vi "Calculate Placing Accuracy.vi"() -> ()   [LabVIEW 2017]
uses:
  Shared Components/Gantry Class/Type Definitions/Virtual Modes.ctl
  Shared Components/Gantry Class/Type Definitions/Init_Modes.ctl
  Shared Components/Utils/Type Definitions/Object Types.ctl
  Shared Components/Config Manager Class/Type Definitions/Camera Enum.ctl
  Shared Components/Gantry Class/Gantry Class.lvclass
  Shared Components/Vec3d Class/Vec3d Class.lvclass
panel:
  in  "Results Folder":path=path "C:/Users/Admin/Gantry Purdue/pixel-gantry-control/Results"
  out "Point being recorded":string="\\P"
  out "Iteration Number":i32
  in  "Virtual Mode":T1=enum."Virtual"
  in  "stop":bool
  out "Image":T2(plugin-control)
  out "error out":errorcluster
  in  "Config Folder":path=path "C:/Users/Admin/Gantry Purdue/pixel-gantry-control/Config"
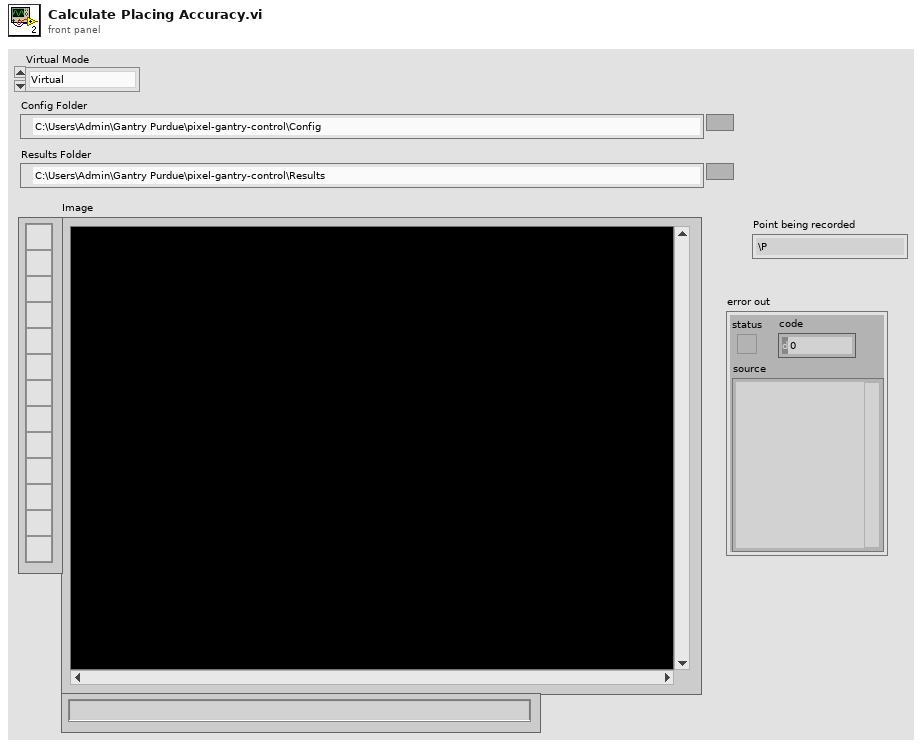
[diagram p1: front panel]
types:
  T1 = typedef "Virtual Modes.ctl" = enum16{"Nonvirtual", "Pseudovirtual", "Virtual"}
  T2 = typedef "IMAQ Image.ctl" = refnum<image>
  T3 = typedef "Init_Modes.ctl" = enum16{"Full", "Robot Only", "Dispenser Only", "Cameras Only", "Robot and Cameras", "Robot and Cameras and Dispenser", "Manifold Only"}
  T4 = typedef "Object Types.ctl" = enum16{"HDI", "Glass Piece", "Other"}
  T5 = typedef "Camera Enum.ctl" = enum16{"GANTRY HEAD", "NEEDLE CALIBRATION X", "NEEDLE CALIBRATION Y", "STAND CAMERA", "SIMRAN WEBCAM"}
  T6 = typedef "Physical Image.ctl" = cluster{"Image Position":refnum<class "Vec3d Class.lvclass">, "Image Reference":T2, "Field of View":cluster{"x(mm)":dbl, "y(mm)":dbl}}
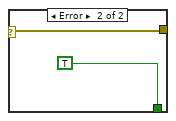
[diagram p2: hidden frame]
diagram:
  n1 = property on="stop" class="Bool (strict)"("Value"=FALSE) -> (error out=w14:errorcluster)  [unwired: 2 in, 1 out]
  n2 = call "IMAQ Create"("Image Name"="test") -> ("New Image"=w11:T2)  [unwired: 4 in, 1 out]
  n3 = property on="error out" class="Clust (strict)"(error in=w14, "Value"=errorcluster {"status"=FALSE, "code"=0, "source"=""} ("error in (no error)")) -> (error out=w9:errorcluster)  [unwired: 1 in, 1 out]
  n4 = call "Create.vi"("Virtual Mode"="Virtual Mode", "error in"=w9, "HOME?"=TRUE, "Config Folder"="Config Folder", "Init Mode"=Init_Modes."Full") -> ("error out"=w6:errorcluster, "Gantry out"=w5:refnum<class "Gantry Class.lvclass">)  [unwired: 5 in]
  n5 = while {
    shift-right: [w72] -> w3
    shift-left: w11 -> [w122]
    shift-right: [w124] -> w2
    shift-left: w5 -> [w158]
    shift-right: [w123] -> w1
    shift-left: w6 -> [w163]
    i -> [w160]
    stop <- w161 stop-if-true
    # "INSERT ROTATION OF STATION"
    # "INSERT MIDPT OF STATION"
    # "Pick up tool"
    # "Return tool"
    n6 = call "HDI fiducials"("error in (no error)"=w163) -> ("error out"=w156:errorcluster)  [unwired: 17 in, 1 out]
    n7 = call-dynamic "Set Manifold Channel.vi"("error in"=w156, "On/Off"=TRUE, "Manifold Channel"=29, "Gantry in"=w158) -> ("error out"=w155:errorcluster, "Gantry out"=w157:refnum<class "Gantry Class.lvclass">)  [unwired: 6 in]
    n8 = call "Create.vi"("error in"=w155, "Z"=30.0, "Y"=193.8, "X"=549.36) -> ("error out"=w243:errorcluster, "Vec3d Class out"=w276:refnum<class "Vec3d Class.lvclass">)  [unwired: 6 in]
    n9 = call-dynamic "Move To Raw.vi"("error in"=w243, "Speed"=80.0, "Destination"=w276, "Gantry in"=w157) -> ("error out"=w63:errorcluster, "Gantry out"=w68:refnum<class "Gantry Class.lvclass">)  [unwired: 6 in]
    n10 = call "Create.vi"("error in"=w63, "Z"=57.76) -> ("error out"=w62:errorcluster, "Vec3d Class out"=w69:refnum<class "Vec3d Class.lvclass">)  [unwired: 8 in]
    n11 = call-dynamic "Move To Raw Relative.vi"("error in"=w62, "Speed(mm/s)"=10.0, "Delta"=w69, "Gantry in"=w68) -> ("error out"=w66:errorcluster, "Gantry out"=w67:refnum<class "Gantry Class.lvclass">)  [unwired: 6 in]
    n12 = call-dynamic "Midpt&Orient.vi"("error in (no error)"=w66, "Enum"=Object_Types."Glass Piece", "Image In"=w122, "Gantry Class in"=w67) -> ("error out"=w176:errorcluster, "Midpoint"=w241:refnum<class "Vec3d Class.lvclass">, "Image Out"=w25:T2, "Gantry Class out"=w168:refnum<class "Gantry Class.lvclass">, "Orientation"=w165:dbl)  [unwired: 3 in]
    n13 = call "Create.vi"("error in"=w176, "Z"=34.374944 ("Y"), "Y"=-101.797103, "X"=-0.484739) -> ("error out"=w169:errorcluster, "Vec3d Class out"=w214:refnum<class "Vec3d Class.lvclass">)  [unwired: 6 in]
    n14 = call-dynamic "Home Single.vi"("error in"=w169, "Axis"=enum16{"X", "Y", "Z", "U"}."Z", "Gantry in"=w168) -> ("error out"=w166:errorcluster, "Gantry out"=w167:refnum<class "Gantry Class.lvclass">)  [unwired: 7 in]
    n15 = call "Create.vi"("error in"=w166, "Y"=16.37, "X"=603.594) -> ("Vec3d Class out"=w292:refnum<class "Vec3d Class.lvclass">)  [unwired: 7 in, 1 out]
    n16 = call-dynamic "Move To Raw.vi"("Speed"=50.0 ("Speed(mm/s)"), "Destination"=w292, "Gantry in"=w167) -> ("error out"=w188:errorcluster, "Gantry out"=w189:refnum<class "Gantry Class.lvclass">)  [unwired: 7 in]
    n17 = call "Create.vi"("Z"=36.7) -> ("Vec3d Class out"=w190:refnum<class "Vec3d Class.lvclass">)  [unwired: 9 in, 1 out]
    n18 = call-dynamic "Move To Raw Relative.vi"("error in"=w188, "Speed(mm/s)"=10.0, "Delta"=w190, "Gantry in"=w189) -> ("error out"=w52:errorcluster, "Gantry out"=w51:refnum<class "Gantry Class.lvclass">)  [unwired: 6 in]
    n19 = call-dynamic "Set Manifold Channel.vi"("error in"=w52, "On/Off"=TRUE, "Manifold Channel"=0, "Gantry in"=w51) -> ("error out"=w54:errorcluster, "Gantry out"=w56:refnum<class "Gantry Class.lvclass">)  [unwired: 6 in]
    n20 = call "Create.vi"("Z"=4.5) -> ("Vec3d Class out"=w57:refnum<class "Vec3d Class.lvclass">)  [unwired: 9 in, 1 out]
    n21 = call-dynamic "Move To Raw Relative.vi"("error in"=w54, "Speed(mm/s)"=1.0, "Delta"=w57, "Gantry in"=w56) -> ("error out"=w53:errorcluster, "Gantry out"=w55:refnum<class "Gantry Class.lvclass">)  [unwired: 6 in]
    n22 = flat-sequence {
      tunnel: w55 -> [w380]
      tunnel: [w380] -> w250
      tunnel: w53 -> [w378]
      tunnel: [w378] -> w249
      frame #0 {
        n23 = Wait (ms)(milliseconds to wait=u32 1000) -> ()  [unwired: 1 out]
      }
    }
    n24 = call "Create.vi"("Z"=-4.5) -> ("Vec3d Class out"=w287:refnum<class "Vec3d Class.lvclass">)  [unwired: 9 in, 1 out]
    n25 = call-dynamic "Move To Raw Relative.vi"("Wait?"=TRUE, "error in"=w249, "Speed(mm/s)"=1.0, "Delta"=w287, "Gantry in"=w250) -> ("error out"=w282:errorcluster, "Gantry out"=w283:refnum<class "Gantry Class.lvclass">)  [unwired: 5 in]
    n26 = call "Create.vi"("Y"=80.0 ("Z")) -> ("Vec3d Class out"=w281:refnum<class "Vec3d Class.lvclass">)  [unwired: 9 in, 1 out]
    n27 = call-dynamic "Move To Raw Relative.vi"("error in"=w282, "Speed(mm/s)"=10.0, "Delta"=w281, "Gantry in"=w283) -> ("error out"=w269:errorcluster, "Gantry out"=w271:refnum<class "Gantry Class.lvclass">)  [unwired: 6 in]
    n28 = call-dynamic "Get Current Position Raw.vi"("error in"=w269, "Gantry in"=w271) -> ("error out"=w268:errorcluster, "Vec3d Class out"=w205:refnum<class "Vec3d Class.lvclass">, "Gantry out"=w270:refnum<class "Gantry Class.lvclass">)  [unwired: 7 in]
    n29 = call "Create.vi"("Z"=-36.7) -> ("Vec3d Class out"=w277:refnum<class "Vec3d Class.lvclass">)  [unwired: 9 in, 1 out]
    n30 = call-dynamic "Move To Raw Relative.vi"("error in"=w268, "Speed(mm/s)"=10.0, "Delta"=w277, "Gantry in"=w270) -> ("error out"=w235:errorcluster, "Gantry out"=w233:refnum<class "Gantry Class.lvclass">)  [unwired: 6 in]
    n31 = call "Subtract Vec3d.vi"("error in (no error)"=w235, "Vec3d in 2"=w214, "Vec3d in 1"=w241) -> ("error out"=w237:errorcluster, "Vec3d Class out"=w194:refnum<class "Vec3d Class.lvclass">)  [unwired: 7 in]
    n32 = call-dynamic "Read Data 2.vi"("error in"=w237, "Vec3d in"=w194) -> ("error out"=w236:errorcluster, "Z"=w39:dbl, "Y"=w239:dbl, "X"=w240:dbl)  [unwired: 6 in]
    n33 = call "Create.vi"("error in"=w236, "Y"=w239, "X"=w240) -> ("error out"=w234:errorcluster, "Vec3d Class out"=w193:refnum<class "Vec3d Class.lvclass">)  [unwired: 7 in]
    n34 = call-dynamic "Move To Raw.vi"("error in"=w234, "Speed"=40.0, "Destination"=w193, "Gantry in"=w233) -> ("error out"=w204:errorcluster, "Gantry out"=w203:refnum<class "Gantry Class.lvclass">)  [unwired: 6 in]
    n35 = call-dynamic "Rotate.vi"("error in"=w204, "speed(deg/s)"=5.0, "distance(deg)"=w165, "Gantry in"=w203) -> ("error out"=w201:errorcluster, "Gantry out"=w202:refnum<class "Gantry Class.lvclass">)  [unwired: 6 in]
    n36 = Subtract(x=w39, y=1.0) -> (x-y=w38:dbl)
    n37 = call "Create.vi"("error in"=w201, "Z"=w38) -> ("error out"=w232:errorcluster, "Vec3d Class out"=w238:refnum<class "Vec3d Class.lvclass">)  [unwired: 8 in]
    n38 = call-dynamic "Move To Raw Relative.vi"("error in"=w232, "Speed(mm/s)"=10.0, "Delta"=w238, "Gantry in"=w202) -> ("error out"=w46:errorcluster, "Gantry out"=w45:refnum<class "Gantry Class.lvclass">)  [unwired: 6 in]
    n39 = call-dynamic "Set Manifold Channel.vi"("error in"=w46, "On/Off"=TRUE, "Manifold Channel"=2, "Gantry in"=w45) -> ("error out"=w48:errorcluster, "Gantry out"=w49:refnum<class "Gantry Class.lvclass">)  [unwired: 6 in]
    n40 = flat-sequence {
      tunnel: w49 -> [w296]
      tunnel: [w296] -> w41
      tunnel: w48 -> [w294]
      tunnel: [w294] -> w34
      frame #0 {
        n41 = Wait (ms)(milliseconds to wait=u32 1500) -> ()  [unwired: 1 out]
      }
    }
    n42 = call "Create.vi"("error in"=w34, "Z"=1.0 ("y")) -> ("error out"=w43:errorcluster, "Vec3d Class out"=w44:refnum<class "Vec3d Class.lvclass">)  [unwired: 8 in]
    n43 = call-dynamic "Move To Raw Relative.vi"("error in"=w43, "Speed(mm/s)"=0.5, "Delta"=w44, "Gantry in"=w41) -> ("error out"=w35:errorcluster, "Gantry out"=w36:refnum<class "Gantry Class.lvclass">)  [unwired: 6 in]
    n44 = call-dynamic "Set Manifold Channel.vi"("error in"=w35, "On/Off"=FALSE, "Manifold Channel"=29, "Gantry in"=w36) -> ("error out"=w151:errorcluster, "Gantry out"=w150:refnum<class "Gantry Class.lvclass">)  [unwired: 6 in]
    n45 = flat-sequence {
      tunnel: w150 -> [w364]
      tunnel: [w364] -> w29
      tunnel: w151 -> [w362]
      tunnel: [w362] -> w28
      frame #0 {
        n46 = Wait (ms)(milliseconds to wait=u32 500) -> ()  [unwired: 1 out]
      }
    }
    n47 = call "Create.vi"("error in"=w28, "Z"=-2.0 ("y")) -> ("error out"=w32:errorcluster, "Vec3d Class out"=w33:refnum<class "Vec3d Class.lvclass">)  [unwired: 8 in]
    n48 = call-dynamic "Move To Raw Relative.vi"("error in"=w32, "Speed(mm/s)"=0.5, "Delta"=w33, "Gantry in"=w29) -> ("error out"=w26:errorcluster, "Gantry out"=w27:refnum<class "Gantry Class.lvclass">)  [unwired: 6 in]
    n49 = Multiply(x=-1.0, y=28.0) -> (x*y=w274:dbl)
    n50 = call "Create.vi"("error in"=w26, "Z"=w274) -> ("error out"=w272:errorcluster, "Vec3d Class out"=w273:refnum<class "Vec3d Class.lvclass">)  [unwired: 8 in]
    n51 = call-dynamic "Move To Raw Relative.vi"("error in"=w272, "Speed(mm/s)"=5.0, "Delta"=w273, "Gantry in"=w27) -> ("error out"=w210:errorcluster, "Gantry out"=w211:refnum<class "Gantry Class.lvclass">)  [unwired: 6 in]
    n52 = call "Create.vi"("Z"=99.68434, "Y"=549.287012, "X"=107.82655) -> ("Vec3d Class out"=w121:refnum<class "Vec3d Class.lvclass">)  [unwired: 7 in, 1 out]
    n53 = call "Subtract Vec3d.vi"("error in (no error)"=w210, "Vec3d in 2"=w214, "Vec3d in 1"=w121) -> ("error out"=w221:errorcluster, "Vec3d Class out"=w224:refnum<class "Vec3d Class.lvclass">)  [unwired: 7 in]
    n54 = Subtract(x=0.0, y=w165) -> (x-y=w164:dbl)
    n55 = call-dynamic "Read Data 2.vi"("error in"=w221, "Vec3d in"=w224) -> ("error out"=w220:errorcluster, "Z"=w112:dbl, "Y"=w225:dbl, "X"=w226:dbl)  [unwired: 6 in]
    n56 = Subtract(x=w112, y=32.0) -> (x-y=w111:dbl)
    n57 = call "Create.vi"("error in"=w220, "Z"=w111, "Y"=w225, "X"=w226) -> ("error out"=w219:errorcluster, "Vec3d Class out"=w223:refnum<class "Vec3d Class.lvclass">)  [unwired: 6 in]
    n58 = call-dynamic "Move To Raw.vi"("error in"=w219, "Speed"=20.0, "Destination"=w223, "Gantry in"=w211) -> ("error out"=w198:errorcluster, "Gantry out"=w199:refnum<class "Gantry Class.lvclass">)  [unwired: 6 in]
    n59 = call-dynamic "Rotate.vi"("error in"=w198, "speed(deg/s)"=5.0, "distance(deg)"=w164, "Gantry in"=w199) -> ("error out"=w197:errorcluster, "Gantry out"=w196:refnum<class "Gantry Class.lvclass">)  [unwired: 6 in]
    n60 = call "Create.vi"("error in"=w197, "Z"=30.0, "Y"=-1.05, "X"=-0.1) -> ("error out"=w218:errorcluster, "Vec3d Class out"=w222:refnum<class "Vec3d Class.lvclass">)  [unwired: 6 in]
    n61 = call-dynamic "Move To Raw Relative.vi"("error in"=w218, "Speed(mm/s)"=5.0, "Delta"=w222, "Gantry in"=w196) -> ("error out"=w19:errorcluster, "Gantry out"=w20:refnum<class "Gantry Class.lvclass">)  [unwired: 6 in]
    n62 = call "Create.vi"("error in"=w19, "Z"=2.0) -> ("error out"=w23:errorcluster, "Vec3d Class out"=w24:refnum<class "Vec3d Class.lvclass">)  [unwired: 8 in]
    n63 = call-dynamic "Move To Raw Relative.vi"("error in"=w23, "Speed(mm/s)"=0.5, "Delta"=w24, "Gantry in"=w20) -> ("error out"=w18:errorcluster, "Gantry out"=w17:refnum<class "Gantry Class.lvclass">)  [unwired: 6 in]
    n64 = call-dynamic "Set Manifold Channel.vi"("error in"=w18, "On/Off"=FALSE, "Manifold Channel"=2, "Gantry in"=w17) -> ("error out"=w213:errorcluster, "Gantry out"=w212:refnum<class "Gantry Class.lvclass">)  [unwired: 6 in]
    n65 = flat-sequence {
      tunnel: w212 -> [w374]
      tunnel: [w374] -> w146
      tunnel: w213 -> [w372]
      tunnel: [w372] -> w143
      frame #0 {
        n66 = Wait (ms)(milliseconds to wait=u32 1500) -> ()  [unwired: 1 out]
      }
    }
    n67 = call-dynamic "Set Manifold Channel.vi"("error in"=w143, "On/Off"=TRUE, "Manifold Channel"=24, "Gantry in"=w146) -> ("error out"=w148:errorcluster, "Gantry out"=w147:refnum<class "Gantry Class.lvclass">)  [unwired: 6 in]
    n68 = flat-sequence {
      tunnel: w147 -> [w361]
      tunnel: [w361] -> w145
      tunnel: w148 -> [w359]
      tunnel: [w359] -> _
      tunnel: [w359] -> w144
      frame #0 {
        n69 = Wait (ms)(milliseconds to wait=u32 1500) -> ()  [unwired: 1 out]
      }
    }
    n70 = Multiply(x=-1.0, y=w112) -> (x*y=w228:dbl)
    n71 = call "Create.vi"("error in"=w144, "Z"=w228) -> ("error out"=w209:errorcluster, "Vec3d Class out"=w206:refnum<class "Vec3d Class.lvclass">)  [unwired: 8 in]
    n72 = call-dynamic "Move To Raw Relative.vi"("error in"=w209, "Delta"=w206, "Gantry in"=w145) -> ("error out"=w207:errorcluster, "Gantry out"=w208:refnum<class "Gantry Class.lvclass">)  [unwired: 7 in]
    n73 = call-dynamic "Move To Raw.vi"("error in"=w207, "Speed"=40.0, "Destination"=w205, "Gantry in"=w208) -> ("error out"=w179:errorcluster, "Gantry out"=w187:refnum<class "Gantry Class.lvclass">)  [unwired: 6 in]
    n74 = call "Create.vi"("error in"=w179, "Y"=-80.0) -> ("error out"=w266:errorcluster, "Vec3d Class out"=w251:refnum<class "Vec3d Class.lvclass">)  [unwired: 8 in]
    n75 = call-dynamic "Move To Raw Relative.vi"("error in"=w266, "Speed(mm/s)"=20.0, "Delta"=w251, "Gantry in"=w187) -> ("error out"=w252:errorcluster, "Gantry out"=w253:refnum<class "Gantry Class.lvclass">)  [unwired: 6 in]
    n76 = call "Create.vi"("Z"=4.5) -> ("Vec3d Class out"=w259:refnum<class "Vec3d Class.lvclass">)  [unwired: 9 in, 1 out]
    n77 = call-dynamic "Move To Raw Relative.vi"("error in"=w252, "Speed(mm/s)"=5.0, "Delta"=w259, "Gantry in"=w253) -> ("error out"=w257:errorcluster, "Gantry out"=w258:refnum<class "Gantry Class.lvclass">)  [unwired: 6 in]
    n78 = call-dynamic "Set Manifold Channel.vi"("error in"=w257, "On/Off"=FALSE, "Manifold Channel"=0, "Gantry in"=w258) -> ("error out"=w246:errorcluster, "Gantry out"=w248:refnum<class "Gantry Class.lvclass">)  [unwired: 6 in]
    n79 = flat-sequence {
      tunnel: w248 -> [w377]
      tunnel: [w377] -> w247
      tunnel: w246 -> [w375]
      tunnel: [w375] -> w245
      frame #0 {
        n80 = Wait (ms)(milliseconds to wait=u32 1500) -> ()  [unwired: 1 out]
      }
    }
    n81 = call "Create.vi"("Z"=-4.5) -> ("Vec3d Class out"=w255:refnum<class "Vec3d Class.lvclass">)  [unwired: 9 in, 1 out]
    n82 = call-dynamic "Move To Raw Relative.vi"("error in"=w245, "Speed(mm/s)"=5.0, "Delta"=w255, "Gantry in"=w247) -> ("error out"=w134:errorcluster, "Gantry out"=w135:refnum<class "Gantry Class.lvclass">)  [unwired: 6 in]
    n83 = call "Create.vi"("Z"=-36.7) -> ("Vec3d Class out"=w137:refnum<class "Vec3d Class.lvclass">)  [unwired: 9 in, 1 out]
    n84 = call-dynamic "Move To Raw Relative.vi"("error in"=w134, "Speed(mm/s)"=50.0, "Delta"=w137, "Gantry in"=w135) -> ("error out"=w125:errorcluster, "Gantry out"=w126:refnum<class "Gantry Class.lvclass">)  [unwired: 6 in]
    n85 = call "Create.vi"("error in"=w125, "Z"=30.0, "Y"=560.0, "X"=120.0) -> ("error out"=w129:errorcluster, "Vec3d Class out"=w131:refnum<class "Vec3d Class.lvclass">)  [unwired: 6 in]
    n86 = call-dynamic "Move To Raw.vi"("error in"=w129, "Speed"=80.0, "Destination"=w131, "Gantry in"=w126) -> ("error out"=w74:errorcluster, "Gantry out"=w75:refnum<class "Gantry Class.lvclass">)  [unwired: 6 in]
    n87 = Build Array("Glass_TL_fiducial" ("string"), "Glass_BL_fidiucial" ("string")) -> (w109:string[])
    n88 = for {
      tunnel: [w350] -> w77 mode=indexing
      shift-right: [w351] -> w98
      shift-left: w74 -> [w335]
      shift-right: [w349] -> w99
      shift-left: w75 -> [w342]
      shift-right: [w343] -> w89
      shift-left: w25 -> [w348]
      tunnel: w109 -> [w345] mode=indexing
      i -> [w332]
      n89 = Index Array(array=dbl[] [99.115052, 99.014207], index=w332) -> (element=w339:dbl)
      n90 = Index Array(array=dbl[] [526.637597, 569.837549], index=w332) -> (element=w338:dbl)
      n91 = call "Create.vi"("error in"=w335, "Z"=99.700001, "Y"=w338, "X"=w339) -> ("error out"=w334:errorcluster, "Vec3d Class out"=w336:refnum<class "Vec3d Class.lvclass">)  [unwired: 6 in]
      n92 = call-dynamic "Move To Raw.vi"("error in"=w334, "Speed"=10.0, "Destination"=w336, "Gantry in"=w342) -> ("error out"=w341:errorcluster, "Gantry out"=w340:refnum<class "Gantry Class.lvclass">)  [unwired: 6 in]
      n93 = call-dynamic "Joystick with Image Update.vi"("error in (no error)"=w341, "Image In"=w348, "Gantry Class in"=w340) -> ("error out"=w358:errorcluster, "Image Out"=w347:T2, "Gantry Class out"=w357:refnum<class "Gantry Class.lvclass">)  [unwired: 6 in]
      n94 = call-dynamic "Get Physical Image.vi"("error in"=w358, "Image In"=w347, "Camera Name"=Camera_Enum."GANTRY HEAD", "Gantry in"=w357) -> ("error out"=w352:errorcluster, "Physical Image"=w356:T6, "Gantry out"=w349:refnum<class "Gantry Class.lvclass">)  [unwired: 5 in]
      n95 = Unbundle By Name(w356) -> ("Image Position"=w355:refnum<class "Vec3d Class.lvclass">, "Image Reference"=w343:T2)
      n96 = call "To String.vi"("error in"=w352, "Vec3d in"=w355) -> ("error out"=w351:errorcluster, "Vec3d String"=w353:string)  [unwired: 7 in, 1 out]
      n97 = Concatenate Strings(w345, ":(" ("string"), w353, ")" ("string"), "\r\n" ("string")) -> (w350:string)
      "Point being recorded" <- w345
    }
    n98 = call-dynamic "Home Single.vi"("error in"=w98, "Axis"=enum16{"X", "Y", "Z", "U"}."Z", "Gantry in"=w99) -> ("error out"=w93:errorcluster, "Gantry out"=w95:refnum<class "Gantry Class.lvclass">)  [unwired: 7 in]
    n99 = call "Create.vi"("error in"=w93, "Y"=-100.0) -> ("error out"=w92:errorcluster, "Vec3d Class out"=w97:refnum<class "Vec3d Class.lvclass">)  [unwired: 8 in]
    n100 = call-dynamic "Move To Raw Relative.vi"("error in"=w92, "Speed(mm/s)"=50.0, "Delta"=w97, "Gantry in"=w95) -> ("error out"=w91:errorcluster, "Gantry out"=w90:refnum<class "Gantry Class.lvclass">)  [unwired: 6 in]
    n101 = call "HDI placement"("error in (no error)"=w91) -> ("error out"=w88:errorcluster)  [unwired: 17 in, 1 out]
    n102 = Build Array("Glass_TR_bondpad" ("string"), "HDI_TR_bondpad" ("string"), "Glass_M1R_bondpad" ("string"), "HDI_M1R_bondpad" ("string"), "Glass_M2R_bondpad" ("string"), "HDI_M2R_bondpad" ("string"), "Glass_BR_bondpad" ("string"), "HDI_BR_bondpad" ("string")) -> (w86:string[])
    n103 = for {
      tunnel: [w321] -> w70 mode=indexing
      shift-right: [w322] -> w87
      shift-left: w88 -> [w301]
      shift-right: [w320] -> w73
      shift-left: w90 -> [w315]
      shift-right: [w316] -> w72
      shift-left: w89 -> [w304]
      tunnel: w86 -> [w298] mode=indexing
      i -> [w297]
      n104 = property on="Point being recorded" class="Str"(error in=w301, "Value"=w298) -> (error out=w300:errorcluster)  [unwired: 1 in, 1 out]
      n105 = Index Array(array=dbl[] [117.865655, 115.865431, 117.81352, 115.825048, 117.810515, 115.816289, 117.764379, 115.772791], index=w297) -> (element=w312:dbl)
      n106 = Index Array(array=dbl[] [527.47805, 528.820699, 547.251419, 548.442631, 549.327934, 550.635586, 569.099929, 570.297009], index=w297) -> (element=w311:dbl)
      n107 = Index Array(array=dbl[] [99.69002, 99.174729, 99.649999, 98.989215, 99.684328, 98.962658, 99.645157, 99.21018], index=w297) -> (element=w302:dbl)
      n108 = call "Create.vi"("error in"=w300, "Z"=w302, "Y"=w311, "X"=w312) -> ("error out"=w309:errorcluster, "Vec3d Class out"=w310:refnum<class "Vec3d Class.lvclass">)  [unwired: 6 in]
      n109 = call-dynamic "Move To Raw.vi"("error in"=w309, "Speed"=10.0, "Destination"=w310, "Gantry in"=w315) -> ("error out"=w314:errorcluster, "Gantry out"=w313:refnum<class "Gantry Class.lvclass">)  [unwired: 6 in]
      n110 = call-dynamic "Joystick with Image Update.vi"("error in (no error)"=w314, "Image In"=w304, "Gantry Class in"=w313) -> ("error out"=w328:errorcluster, "Image Out"=w319:T2, "Gantry Class out"=w327:refnum<class "Gantry Class.lvclass">)  [unwired: 6 in]
      n111 = call-dynamic "Get Physical Image.vi"("error in"=w328, "Image In"=w319, "Camera Name"=Camera_Enum."GANTRY HEAD", "Gantry in"=w327) -> ("error out"=w299:errorcluster, "Physical Image"=w326:T6, "Gantry out"=w320:refnum<class "Gantry Class.lvclass">)  [unwired: 5 in]
      n112 = Unbundle By Name(w326) -> ("Image Position"=w325:refnum<class "Vec3d Class.lvclass">, "Image Reference"=w316:T2)
      n113 = call "To String.vi"("error in"=w299, "Vec3d in"=w325) -> ("error out"=w322:errorcluster, "Vec3d String"=w323:string)  [unwired: 7 in, 1 out]
      n114 = Concatenate Strings(w298, ":(" ("string"), w323, ")" ("string"), "\r\n" ("string")) -> (w321:string)
    }
    n115 = Format Date/Time String(time format string (%c)="%d%b%y_%H-%M") -> (date/time string=w102:string)  [unwired: 2 in]
    n116 = Concatenate Strings(w77, w70) -> (w76:string)
    n117 = Concatenate Strings("Accuracy_DataPoint_Glass_" ("name or relative path"), w102, ".txt" ("string")) -> (w104:string)
    n118 = Build Path(base path="Results Folder", name or relative path=w104) -> (appended path=w107:path)
    n119 = Write to Text File(file (use dialog)=w107, text=w76, error in=w87) -> (error out=w71:errorcluster)  [unwired: 1 in, 2 out]
    n120 = call-dynamic "Set Manifold Channel.vi"("error in"=w71, "On/Off"=FALSE, "Manifold Channel"=24, "Gantry in"=w73) -> ("error out"=w139:errorcluster, "Gantry out"=w138:refnum<class "Gantry Class.lvclass">)  [unwired: 6 in]
    n121 = call-dynamic "Home Single.vi"("error in"=w139, "Axis"=enum16{"X", "Y", "Z", "U"}."Z", "Gantry in"=w138) -> ("error out"=w182:errorcluster, "Gantry out"=w183:refnum<class "Gantry Class.lvclass">)  [unwired: 7 in]
    n122 = call-dynamic "Home Single.vi"("error in"=w182, "Axis"=enum16{"X", "Y", "Z", "U"}."Y", "Gantry in"=w183) -> ("error out"=w180:errorcluster, "Gantry out"=w181:refnum<class "Gantry Class.lvclass">)  [unwired: 7 in]
    n123 = call-dynamic "Home Single.vi"("error in"=w180, "Axis"=enum16{"X", "Y", "Z", "U"}."X", "Gantry in"=w181) -> ("error out"=w162:errorcluster, "Gantry out"=w124:refnum<class "Gantry Class.lvclass">)  [unwired: 7 in]
    n124 = case shown="No Error" w162 {
      selector: w162 -> [w365 w371]
      tunnel: [w365 w371] -> w123
      tunnel: [w366 TRUE ("Done Testing?")] -> w161
      frame No Error {
        n125 = Two Button Dialog(message="Done Testing?", 1:"No" ("F button name (\"Cancel\")"), 2:"Yes" ("T button name (\"OK\")")) -> (T button?=w366:bool)
      }
      frame Error {
      }
    }
    "Iteration Number" <- w160
  }
  n126 = while {
    tunnel: w11 -> [w383]
    stop <- "stop" stop-if-true
    n127 = call "Superimpose Crosshairs.vi"("Grid Line Color"=u32 65518, "Refnum in"=w383) -> ("Refnum out"=→"Image":T2)
    n128 = Wait (ms)(milliseconds to wait=u32 100) -> ()  [unwired: 1 out]
  }
  n129 = call "Destroy.vi"("error in"=w1, "Gantry Class in"=w2) -> ("error out"=→"error out":errorcluster)  [unwired: 9 in]
  n130 = call "IMAQ Dispose"("Image"=w3) -> ()  [unwired: 5 in, 1 out]
